vi "Connection Reader.vi"(8 "error in (no error)":errorcluster, 11 "Network Sink Endpoint in":refnum<class "Network Sink Endpoint.lvclass">) -> (0 "error out":errorcluster, 2 "Stop?":bool, 3 "Network Sink Endpoint out":refnum<class "Network Sink Endpoint.lvclass">)   [LabVIEW 2017, in "Network Sink.lvlib" / "Network Sink Endpoint.lvclass"]
uses:
  <vilib>/gpm_packages/@cs/event-logger/Source/Network Sink/Network Sink Endpoint/Network Sink Endpoint.lvclass
  <vilib>/gpm_packages/@cs/event-logger/Source/Network Sink/Network Sink Endpoint/Network Sink Endpoint.lvclass/Network Sink Endpoint.ctl
  <vilib>/gpm_packages/@cs/event-logger/Source/Composed Log/LoggerReference/LoggerReference.lvclass/LoggerReference.ctl
  <vilib>/gpm_packages/@cs/event-logger/Source/Composed Log/LoggerReference/Log.vi
  <vilib>/gpm_packages/@cs/event-logger/Source/Composed Log/LoggerReference/Get Valid Event Time.vi
  <vilib>/gpm_packages/@cs/event-logger/Source/Composed Log/LoggerReference/Remove Stale Logs.vi
  <vilib>/gpm_packages/@cs/event-logger/Source/Composed Log/LoggerReference/LoggerReference.lvclass
  <vilib>/gpm_packages/@cs/Network-Sink/Source/Network Interface/Network Interface/Network Interface.lvclass
  <vilib>/gpm_packages/@cs/event-logger/Source/Network Sink/LogEventMessageProtocol/LogEventMessageProtocol.lvclass
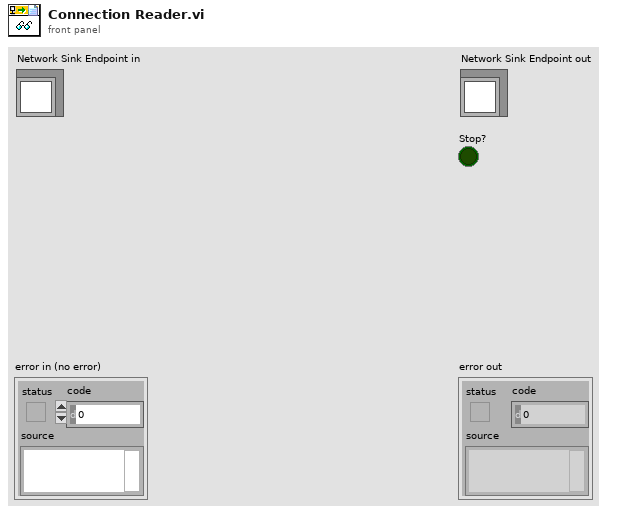
[diagram p1: front panel]
types:
  T1 = typedef "Composed Log.lvlib/Log Packet.ctl" = cluster{"Data To Log":string, "Source":string, "Event Level":T2, "Event Time":timestamp}
  T2 = typedef "Composed Log.lvlib/Log Level.ctl" = enum16{"Debug", "Info", "Warning", "Error", "Critical"}
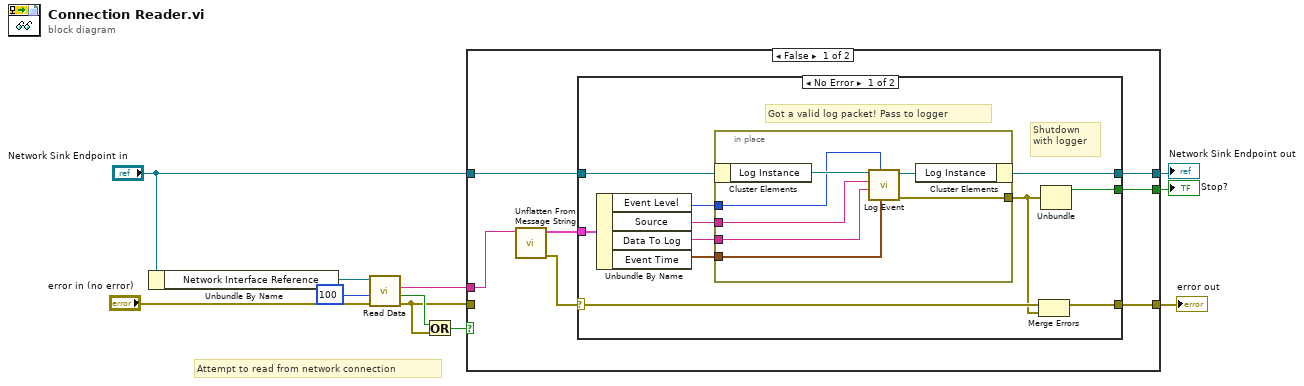
[diagram p0: block diagram]
diagram:
  # "Attempt to read from network connection"
  n1 = Unbundle By Name("Network Sink Endpoint in") -> ("Network Interface Reference"=w9:refnum<data-value>)
  n2 = call <vilib>:"Read Data.vi"("error in (no error)"="error in (no error)", "Timeout in ms (-1)"=100 ("Timeout (ms)"), "Network Interface"=w9) -> ("error out"=w3:errorcluster, "Timed Out?"=w4:bool, "Read Data"=w5:string)  [unwired: 5 in, 1 out]
  n3 = Or(x=w4, y=w3) -> (x .or. y?=w2:bool)
  n4 = case shown="False" w2 {
    tunnel: "Network Sink Endpoint in" -> [w18 w40]
    tunnel: [w17 w40] -> w11
    tunnel: [w16 w39] -> w10
    tunnel: w5 -> [w15 _]
    tunnel: w3 -> [_ w39]
    tunnel: [w12 _] -> w1
    frame False {
      n5 = call <vilib>:"Unflatten From Message String.vi"("Message"=w15) -> ("error out"=w13:errorcluster, "Log Packet"=w14:T1)  [unwired: 9 in]
      n6 = case shown="No Error" w13 {
        selector: w13 -> [w21 w37]
        tunnel: w18 -> [w29 w38]
        tunnel: [w28 w38] -> w17
        tunnel: [w23 w37] -> w16
        tunnel: w14 -> [w22 _]
        tunnel: [w19 _] -> w12
        frame No Error {
          # "Got a valid log packet! Pass to logger"
          # "Shutdown with logger"
          n7 = Unbundle By Name(w22) -> ("Event Level"=w27:T2, "Source"=w26:string, "Data To Log"=w25:string, "Event Time"=w24:timestamp)
          n8 = in-place {
            in-place-border: w27 -> [w34]
            in-place-border: w26 -> [w31]
            in-place-border: w25 -> [w33]
            in-place-border: w24 -> [w30]
            in-place-border: [w32] -> w20
            n9 = in-place-cluster #1(w29) -> ("Log Instance"=w36:refnum<class "LoggerReference.lvclass">)
            n10 = call <vilib>:"Log Event.vi"("Event Time"=w30, "Event Level"=w34, "Data To Log"=w33, "SourceID"=w31, "Log Instance"=w36) -> ("error out"=w32:errorcluster, "Log Instance Out"=w35:refnum<class "LoggerReference.lvclass">)  [unwired: 5 in]
            n11 = in-place-cluster #1("Log Instance"=w35) -> (w28:refnum<class "Network Sink Endpoint.lvclass">)
          }
          n12 = Merge Errors(w21, w20) -> (w23:errorcluster)
          n13 = Unbundle(w20) -> ("status"=w19:bool)  [unwired: 2 out]
        }
        frame Error {
        }
      }
    }
    frame True {
    }
  }
  "error out" <- w10
  "Network Sink Endpoint out" <- w11
  "Stop?" <- w1
